vi "instr.Multimeter_34401A.vi"(7 "timeout (10sec)":u32=2000 caption="超时（10秒）", 8 "error in (no error)":errorcluster caption="错误输入（无错误）", 10 "写入缓冲区":string, 11 "VISA resource name":refnum<visa-resource-name> caption="VISA资源名称") -> (0 "错误输出":errorcluster, 3 "OK?":bool)   [LabVIEW 2012, in "Lib_UEL.ATE.lvlib" / "Lib_Instrument.lvlib"]
uses:
  <vilib>/Instr/_visa.llb/VISA Configure Serial Port (Instr).vi
  Lib_Instrument.lvlib
panel:
  out "返回数":u32
  in  "字节总数":u32
  out "读取缓冲区":string
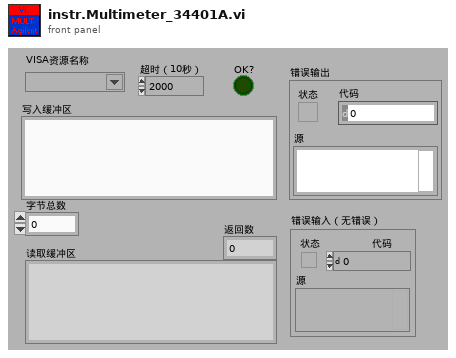
[diagram p1: front panel]
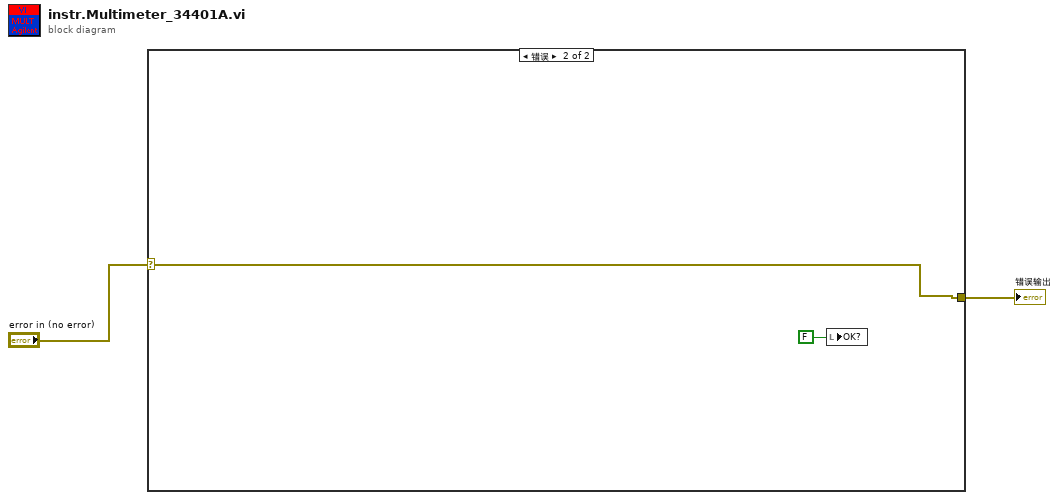
[diagram p0: block diagram]
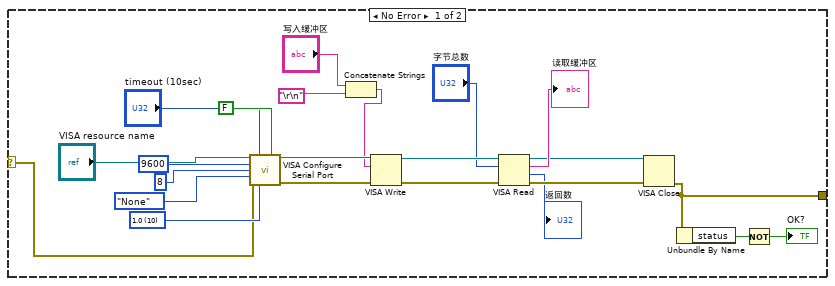
[diagram p2: hidden frame]
diagram:
  n1 = case shown="错误" "error in (no error)" {
    selector: "error in (no error)" -> [w6 w27]
    tunnel: [w5 w27] -> w2
    frame No Error {
      w20 = u16 10 items=["1.0"=10, "1.5"=15, "2.0"=20] ("stop bits (10: 1 bit)")
      n2 = call-poly "VISA Configure Serial Port"("VISA resource name"="VISA resource name", "timeout (10sec)"="timeout (10sec)", "Enable Termination\nChar (T)"=FALSE ("Enable Termination\nChar (T)"), "baud rate (9600)"=u32 9600, "data bits (8)"=u16 8, "parity (0:none)"=enum16{"None", "Odd", "Even", "Mark", "Space"}."None", "error in (no error)"=w6, "stop bits (10: 1 bit)"=w20) -> ("VISA resource name out"=w18:refnum<visa-resource-name>, "error out"=w17:errorcluster)  [unwired: 6 in]
      n3 = Concatenate Strings("写入缓冲区", "\r\n") -> (w7:string)
      n4 = VISA Write(VISA resource name=w18, write buffer=w7, error in (no error)=w17) -> (VISA resource name out=w16:refnum<visa-resource-name>, error out=w15:errorcluster)  [unwired: 1 out]
      n5 = VISA Read(VISA resource name=w16, byte count="字节总数", error in (no error)=w15) -> (VISA resource name out=w12:refnum<visa-resource-name>, read buffer=→"读取缓冲区":string, return count=→"返回数":u32, error out=w11:errorcluster)
      n6 = VISA Close(VISA resource name=w12, error in (no error)=w11) -> (error out=w5:errorcluster)
      n7 = Unbundle By Name(w5) -> ("status"=w4:bool)
      n8 = Not(x=w4) -> (.not. x?=→"OK?":bool)
    }
    frame Error {
      n9 = local write "OK?"(FALSE ("OK?")) -> ()
    }
  }
  "错误输出" <- w2
